vi "P1E2 RLJ 2015640305.vi"() -> ()   [LabVIEW 2016]
panel:
  out "Cluster 3":T1
  out "Cluster 2":T1
  in  "B6":bool
  in  "B0":bool
  in  "B1":bool
  in  "B2":bool
  in  "B3":bool
  in  "B4":bool
  in  "B5":bool
  out "Cluster":T1
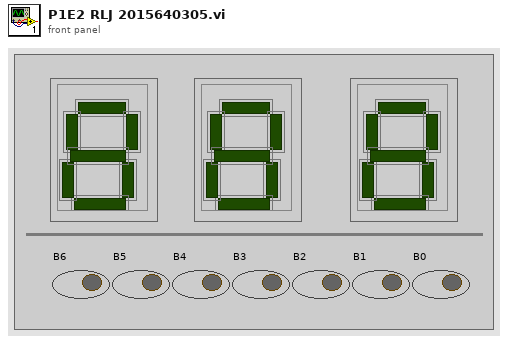
[diagram p1: front panel]
types:
  T1 = cluster{"A":bool, "B":bool, "C":bool, "E":bool, "D":bool, "F":bool, "G":bool}
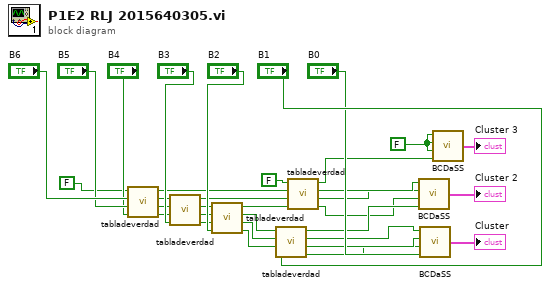
[diagram p0: block diagram]
diagram:
  w1 = FALSE
  n1 = call "tabladeverdad.vi"("Z"="B4", "Y"="B5", "X"="B6", "W"=FALSE) -> ("D"=w17:bool, "C"=w18:bool, "B"=w19:bool, "A"=w16:bool)
  n2 = call "tabladeverdad.vi"("Z"="B3", "Y"=w17, "X"=w18, "W"=w19) -> ("D"=w21:bool, "C"=w22:bool, "B"=w23:bool, "A"=w20:bool)
  n3 = call "tabladeverdad.vi"("Z"="B2", "Y"=w21, "X"=w22, "W"=w23) -> ("D"=w27:bool, "C"=w28:bool, "B"=w29:bool, "A"=w26:bool)
  n4 = call "tabladeverdad.vi"("Z"="B1", "Y"=w27, "X"=w28, "W"=w29) -> ("D"=w7:bool, "C"=w8:bool, "B"=w9:bool, "A"=w6:bool)
  n5 = call "tabladeverdad.vi"("Z"=w26, "Y"=w20, "X"=w16, "W"=FALSE) -> ("D"=w3:bool, "C"=w4:bool, "B"=w5:bool, "A"=w2:bool)
  n6 = call "BCDaSS.vi"("D"=w6, "C"=w3, "B"=w4, "A"=w5) -> ("display"=→"Cluster 2":T1)
  n7 = call "BCDaSS.vi"("D"="B0", "C"=w7, "B"=w8, "A"=w9) -> ("display"=→"Cluster":T1)
  n8 = call "BCDaSS.vi"("D"=w2, "C"=w1, "B"=w1, "A"=w1) -> ("display"=→"Cluster 3":T1)
